vi "Create Response.vi"(6 "id":string, 8 "error in (no error)":errorcluster, 9 "result":variant, 11 "JSON-RPC in":refnum<class "JSON-RPC.lvclass">) -> (0 "error out":errorcluster, 2 "<JSON> Response":string, 3 "JSON-RPC out":refnum<class "JSON-RPC.lvclass">)   [LabVIEW 2019, in "JSON-RPC.lvclass"]
doc: "Format a Response object sent by a Server.\n\n<b>result</b> is a Structured value. The object will be formatted as follows (same as Request params):\n- Clusters will be flattened to json by-name\n- Arrays will be converted to json array\n- Elements (string, float, etc) will be converted to a 1 element json array\n\n<b>id</b> must be the same as the id of the Request Object\n\nhttps://www.jsonrpc.org/specification"
uses:
  JSON-RPC.lvclass
  <vilib>/JDP Science/JSONtext/Make JSON Object.vi
  private/Create Response-JSONtext.vi/8b9e59fa-9ebd-4504-a939-6047597c77d3.vi
  private/Create Error Object.vi
  private/Variant to JSON.vi
  <vilib>/JDP Science/JSONtext/support/Format JSON Object.vi
  <vilib>/JDP Science/JSONtext/Variant to JSON Text.vi
  <vilib>/JDP Science/JSONtext/LVClass Serializer/JSONtext LVClass Serializer.lvclass
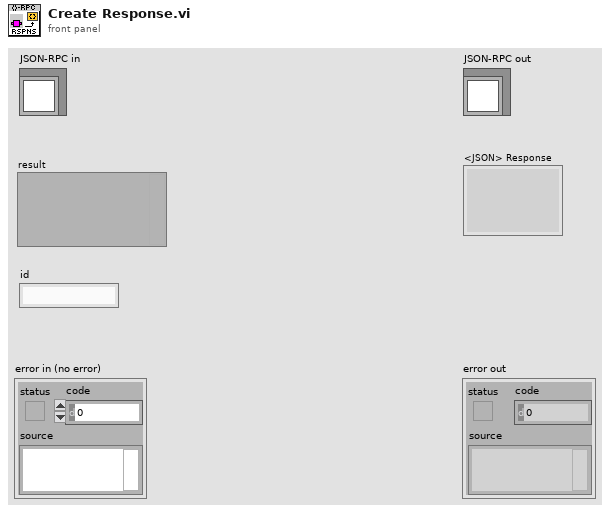
[diagram p1: front panel]
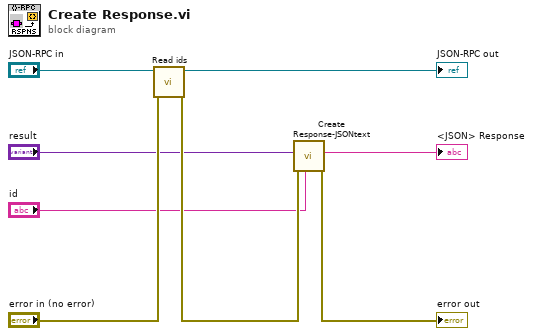
[diagram p0: block diagram]
diagram:
  n1 = call "Read ids.vi"("error in (no error)"="error in (no error)", "JSON-RPC in"="JSON-RPC in") -> ("error out"=w5:errorcluster, "JSON-RPC out"=→"JSON-RPC out":refnum<class "JSON-RPC.lvclass">)  [unwired: 7 in, 1 out]
  n2 = call "Create Response-JSONtext.vi"("id"="id", "error in (no error)"=w5, "result"="result") -> ("error out"=→"error out":errorcluster, "<JSON>"=→"<JSON> Response":string)  [unwired: 7 in]
